vi "VariantToMap.vi"(8 "error in (no error)":errorcluster, 11 "Map":variant) -> (0 "error out":errorcluster, 1 "DecomposedMap":T1[](array[typedef]), 2 "Type":string, 3 "Value":string)   [LabVIEW 2019, in "BlueVariantView.lvlib"]
uses:
  BlueVariantView.lvlib
  DecomposedMap.ctl
  <vilib>/PNR/LabVIEW Composition/Composition/Composition.lvlib
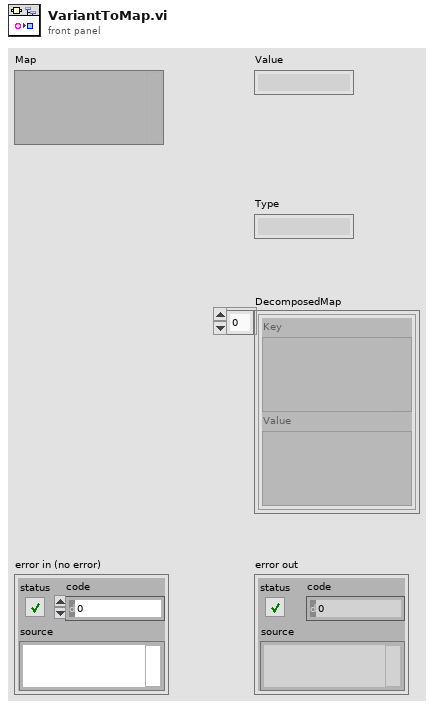
[diagram p1: front panel]
types:
  T1 = typedef "BlueVariantView.lvlib/DecomposedMap.ctl" = cluster{"Key":variant, "Value":variant}
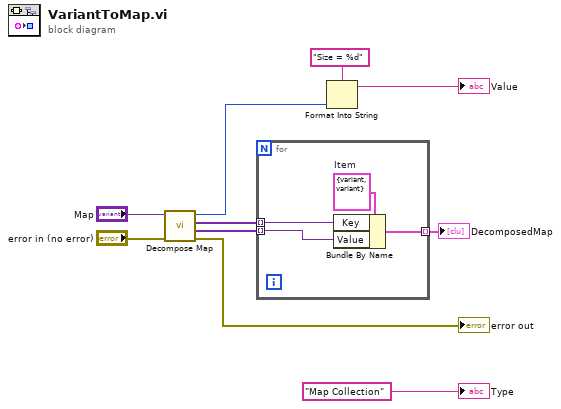
[diagram p0: block diagram]
diagram:
  n1 = call <vilib>:"Decompose Map.vi"("error in (no error)"="error in (no error)", "Variant"="Map") -> ("error out"=→"error out":errorcluster, "Values"=w3:variant[], "Keys"=w4:variant[], "Size"=w5:i32)  [unwired: 6 in]
  n2 = for {
    tunnel: [w14] -> w2 mode=indexing
    tunnel: w4 -> [w12] mode=indexing
    tunnel: w3 -> [w11] mode=indexing
    w13 = T1 {"Key"=variant, "Value"=variant}  # Item
    n3 = Bundle By Name(cluster=w13, "Key"=w12, "Value"=w11) -> (w14:T1)
  }
  "DecomposedMap" <- w2
  n4 = Format Into String(format string="Size = %d", w5) -> (resulting string=→"Value":string)  [unwired: 2 in, 1 out]
  "Type" <- "Map Collection" ("Type")
